vi "Read.Data.vi"(8 "error in (no error)":errorcluster, 10 "timeout ms":i32=100, 11 "Ref":refnum<data-value>) -> (0 "error out":errorcluster, 1 "Timeout?":bool, 2 "Values":dbl[](array[numeric]))   [LabVIEW 2015, in "Data Access API.lvlib" / "Data Access API.lvclass"]
uses:
  Data Access API.lvclass
  Data/Read/Read.lvclass
  Data/Read/Read.lvclass/Read.ctl
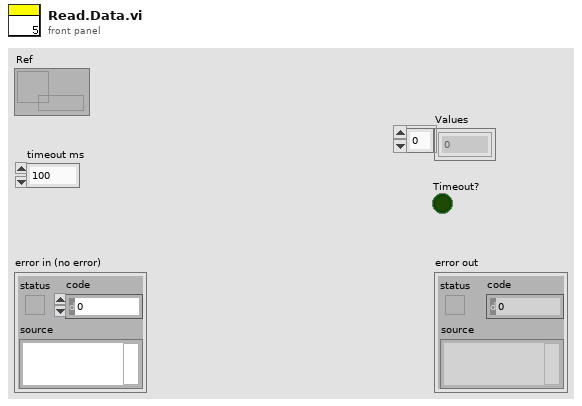
[diagram p1: front panel]
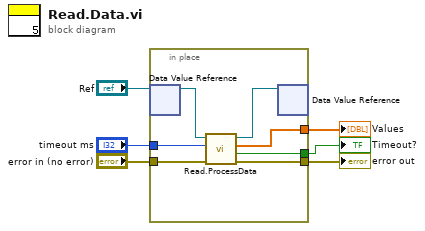
[diagram p0: block diagram]
diagram:
  n1 = in-place {
    in-place-border: "error in (no error)" -> [w13]
    in-place-border: [w12] -> w5
    in-place-border: [w9] -> w3
    in-place-border: "timeout ms" -> [w8]
    in-place-border: [w7] -> w1
    n2 = in-place-dvr #1("Ref") -> (w11:refnum<class "Read.lvclass">)  [unwired: 1 out]
    n3 = call "Read.ProcessData.vi"("error in (no error)"=w13, "timeout ms"=w8, "Read in"=w11) -> ("error out"=w12:errorcluster, "Timeout?"=w7:bool, "Data"=w9:dbl[], "Read out"=w10:refnum<class "Read.lvclass">)  [unwired: 5 in]
    n4 = in-place-dvr #1(w10) -> ()  [unwired: 2 out]
  }
  "error out" <- w5
  "Values" <- w3
  "Timeout?" <- w1
